vi "PlcInfo.vi"() -> ()   [LabVIEW 2018]
uses:
  lib/Snap7.lvlib
panel:
  out "?":string
  out "V3":u8
  out "V2":u8
  out "V1":u8
  out "OrderCode":string
  out "Max MPI Rate":i32
  out "Max Bus Rate":i32
  out "Max Connections":i32
  out "Max PDU Length":i32
  out "Status":string
  out "Result":i32
  out "Module Name":string
  out "Copyright":string
  out "AS Name":string
  out "Serial Number":string
  out "Module Type Name":string
  in  "Slot":i32=2
  in  "Rack":i32
  in  "Address IP":string="192.168.1.12"
  # "Order Code"
  # "V"
  # "CPU Info"
  # "CPU Info"
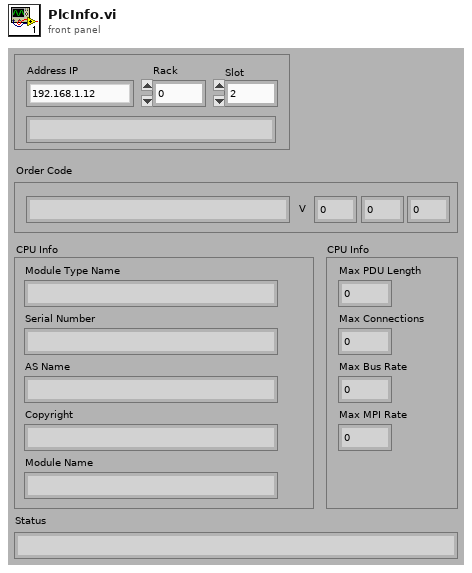
[diagram p1: front panel]
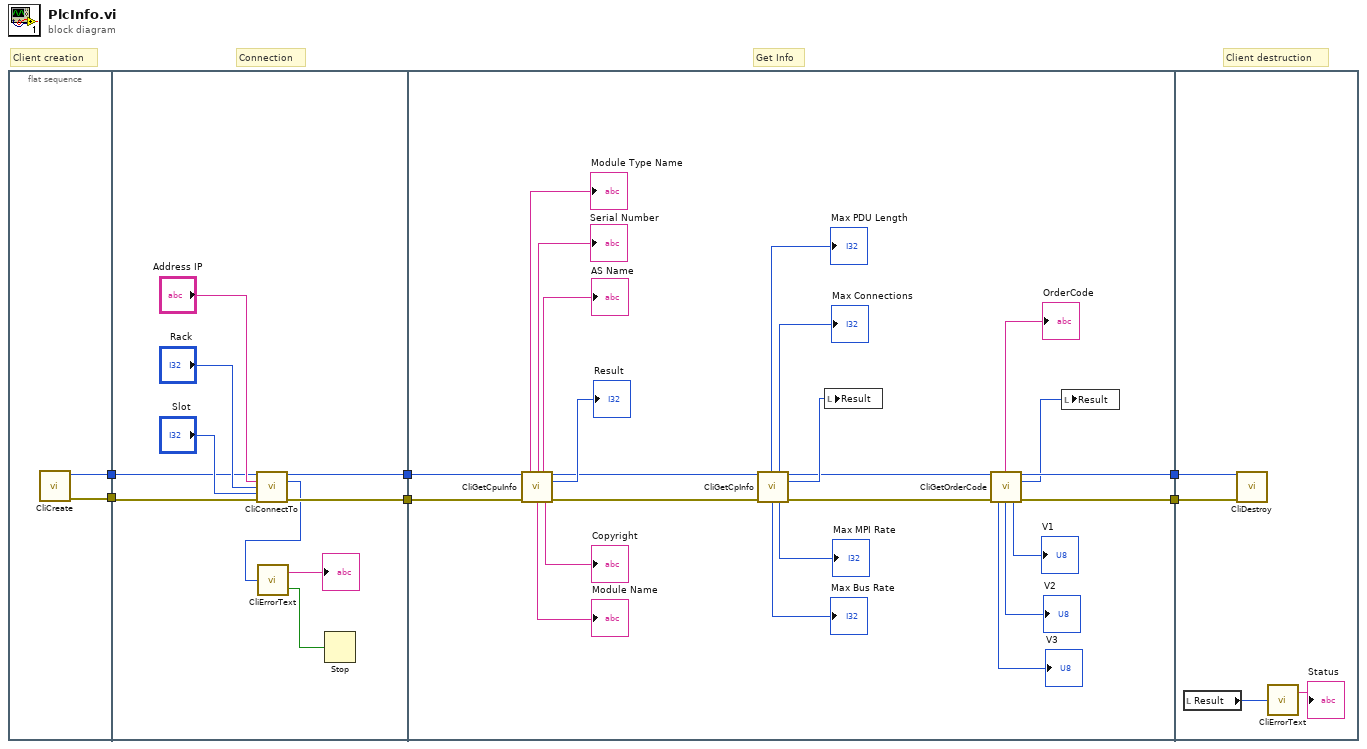
[diagram p0: block diagram]
diagram:
  # "Get Info"
  # "Client destruction"
  # "Connection"
  # "Client creation"
  n1 = flat-sequence {
    tunnel: [w8] -> w4
    tunnel: [w7] -> w3
    tunnel: [w18] -> w6
    tunnel: [w12] -> w5
    tunnel: w4 -> [w14]
    tunnel: w3 -> [w13]
    tunnel: w6 -> [w42]
    tunnel: w5 -> [w41]
    tunnel: [w40] -> w2
    tunnel: [w39] -> w1
    tunnel: w2 -> [w44]
    tunnel: w1 -> [w43]
    frame #0 {
      n2 = call "CliCreate.vi"() -> ("ref out"=w8:u64, "error out"=w7:errorcluster)  [unwired: 14 in]
    }
    frame #1 {
      n3 = call "CliConnectTo.vi"("ref in"=w14, "Address"="Address IP", "Rack"="Rack", "Slot"="Slot", "error in (no error)"=w13) -> ("ref out"=w12:u64, "Result"=w10:i32, "error out"=w18:errorcluster)  [unwired: 8 in]
      n4 = call "CliErrorText.vi"("ErrNo"=w10) -> ("Error"=w11:bool, "ErrMessage"=→"?":string)
      n5 = Stop(stop? (T)=w11) -> ()
    }
    frame #2 {
      n6 = call "CliGetCpuInfo.vi"("ref in"=w41, "error in (no error)"=w42) -> ("ModuleTypeName"=→"Module Type Name":string, "SerialNumber"=→"Serial Number":string, "ASName"=→"AS Name":string, "ref out"=w32:u64, "Result"=→"Result":i32, "ModuleName"=→"Module Name":string, "Copyright"=→"Copyright":string, "error out"=w31:errorcluster)  [unwired: 6 in]
      n7 = call "CliGetCpInfo.vi"("ref in"=w32, "error in (no error)"=w31) -> ("Max PDULength"=→"Max PDU Length":i32, "Max Connections"=→"Max Connections":i32, "ref out"=w25:u64, "Result"=w30:i32, "MaxBus Rate"=→"Max Bus Rate":i32, "Max MPI Rate"=→"Max MPI Rate":i32, "error out"=w24:errorcluster)  [unwired: 7 in]
      n8 = local write "Result"(w30) -> ()
      n9 = call "CliGetOrderCode.vi"("ref in"=w25, "error in (no error)"=w24) -> ("OrderCode"=→"OrderCode":string, "ref out"=w40:u64, "Result"=w22:i32, "V3"=→"V3":u8, "V2"=→"V2":u8, "V1"=→"V1":u8, "error out"=w39:errorcluster)  [unwired: 7 in]
      n10 = local write "Result"(w22) -> ()
    }
    frame #3 {
      n11 = local read "Result"() -> (w45:i32)
      n12 = call "CliDestroy.vi"("ref in"=w44, "error in (no error)"=w43) -> ()  [unwired: 13 in, 1 out]
      n13 = call "CliErrorText.vi"("ErrNo"=w45) -> ("ErrMessage"=→"Status":string)  [unwired: 1 out]
    }
  }
